vi "mass_addressing.vi"(11 "addressings":T1[](array[typedef])) -> (3 "addressing_numeric":u32[](array[numeric]))   [LabVIEW 2014, in "Driver_interaction.lvlib" / "Dali_usb_tridonics.lvclass"]
uses:
  Dali_usb_tridonics.lvclass
  Vendor/Controls/Addressing_type.ctl
  Vendor/Dali_usb.lvlib
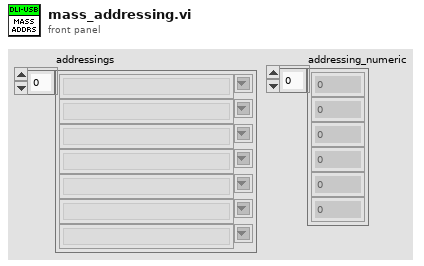
[diagram p1: front panel]
types:
  T1 = typedef "Dali_usb.lvlib/Addressing_type.ctl" = string
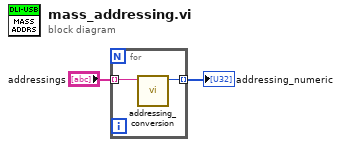
[diagram p0: block diagram]
diagram:
  n1 = for {
    tunnel: "addressings" -> [w4] mode=indexing
    tunnel: [w3] -> w1 mode=indexing
    n2 = call "addressing_conversion.vi"("addressing_type"=w4) -> ("addressing_number"=w3:u32)  [unwired: 10 in]
  }
  "addressing_numeric" <- w1
